vi "classify error.vi"(8 "error to classify":errorcluster, 11 "fixed channel runtime in":refnum<class "CentralErrorHandler runtime.lvclass">) -> (0 "classified error":errorcluster, 2 "error classification":T1, 3 "fixed channel runtime out":refnum<class "CentralErrorHandler runtime.lvclass">)   [LabVIEW 2017, in "CentralErrorHandler runtime.lvclass"]
doc: "Allows a module to classify an error generated at any point during execution. This <b>error classification</b> can then be used by calling code to determine if execution can continue. In addition, this function can be used to allow a component to clear an error, convert an error to a warning, or attempt to recover from an error. Recovery may be attempted only if <b>attempt recovery?</b> is true."
uses:
  CentralErrorHandler runtime.lvclass
  <vilib>/NI/Tag Bus Module Framework/runtime/error classification.ctl
  <vilib>/NI/Tag Bus Module Framework/runtime/TBM module execution interface.lvclass
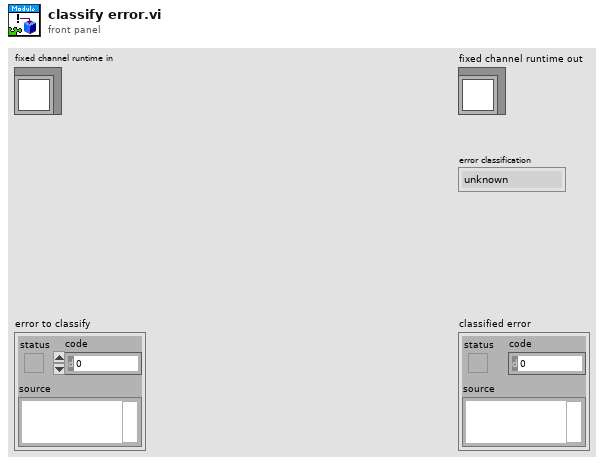
[diagram p1: front panel]
types:
  T1 = typedef "TBM module execution interface.lvclass/error classification.ctl" = enum16{"unknown", "none", "trivial", "recoverable", "critical"}
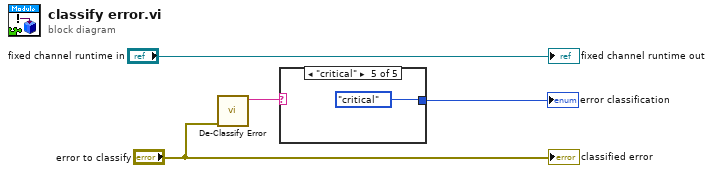
[diagram p0: block diagram]
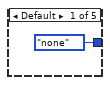
[diagram p2: hidden frame]
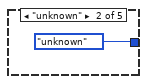
[diagram p3: hidden frame]
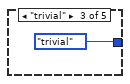
[diagram p4: hidden frame]
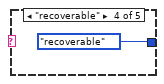
[diagram p5: hidden frame]
diagram:
  n1 = call <userlib>:"De-Classify Error.vi"("Classified Error"="error to classify") -> ("Error Classification"=w2:string)  [unwired: 8 in, 2 out]
  n2 = case shown="\"critical\"" w2 {
    tunnel: [error_classification."none" ("error classification") error_classification."unknown" ("error classification") error_classification."trivial" ("error classification") error_classification."recoverable" ("error classification") error_classification."critical" ("error classification")] -> w1
    frame Default {
    }
    frame "unknown" {
    }
    frame "trivial" {
    }
    frame "recoverable" {
    }
    frame "critical" {
    }
  }
  "error classification" <- w1
  "fixed channel runtime out" <- "fixed channel runtime in"
  "classified error" <- "error to classify"
